vi "Tree_navigation.vi"(8 "error in (no error)":errorcluster, 9 "Tag":string, 10 "Operation":T1(ring), 11 "Script_Tree":refnum<vi>) -> (0 "error out":errorcluster, 2 "Data":string, 3 "Script_Tree 2":refnum<vi>)   [LabVIEW 2024, in "Setting_Screen.lvlib"]
uses:
  Setting_Screen.lvlib
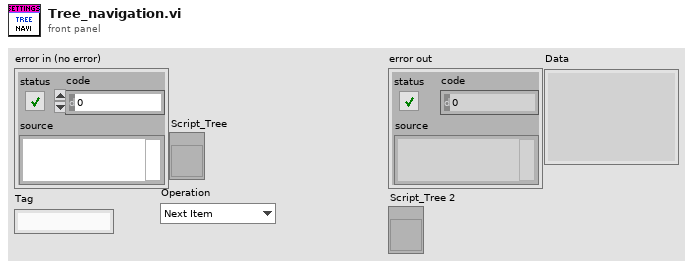
[diagram p1: front panel]
types:
  T1 = enum16{"Next Item", "Previous Item", "Get Child", "Get Parent", "Get Path"}
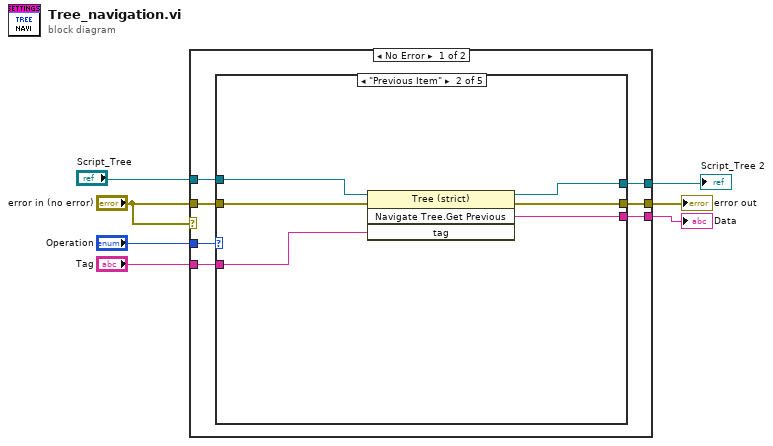
[diagram p0: block diagram]
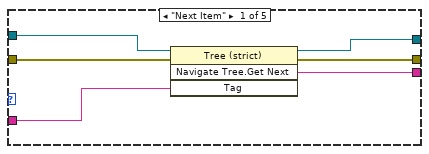
[diagram p2: hidden frame]
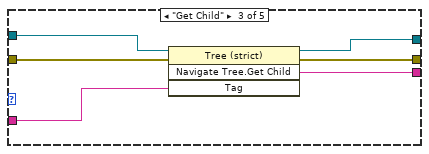
[diagram p3: hidden frame]
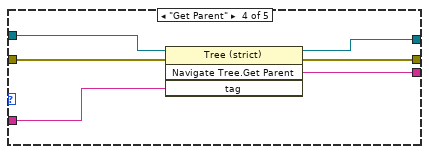
[diagram p4: hidden frame]
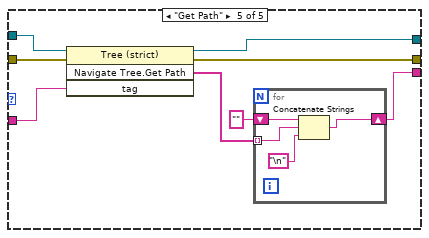
[diagram p5: hidden frame]
diagram:
  n1 = case shown="No Error" "error in (no error)" {
    tunnel: "Operation" -> [w14 _]
    tunnel: "error in (no error)" -> [w13 w51]
    tunnel: "Script_Tree" -> [w12 w52]
    tunnel: [w11 w51] -> w6
    tunnel: [w10 w52] -> w1
    tunnel: [w9 _] -> w5
    tunnel: "Tag" -> [w8 _]
    frame No Error {
      n2 = case shown="\"Previous Item\"" w14 {
        tunnel: w13 -> [w20 w26 w32 w38 w46]
        tunnel: w12 -> [w19 w25 w31 w37 w45]
        tunnel: [w18 w24 w30 w36 w44] -> w10
        tunnel: [w17 w23 w29 w35 w43] -> w11
        tunnel: [w16 w22 w28 w34 w39] -> w9
        tunnel: w8 -> [w15 w21 w27 w33 w42]
        frame "Next Item" {
          n3 = invoke class="Tree (strict)" method="Navigate Tree.Get Next"(reference=w19, error in=w20, "Tag"=w15) -> (reference out=w18:refnum<vi>, error out=w17:errorcluster, "Navigate Tree:Get Next Item"=w16:string)  [unwired: 1 in, 1 out]
        }
        frame "Previous Item" {
          n4 = invoke class="Tree (strict)" method="Navigate Tree.Get Previous"(reference=w25, error in=w26, "tag"=w21) -> (reference out=w24:refnum<vi>, error out=w23:errorcluster, "Navigate Tree:Get Previous"=w22:string)  [unwired: 1 in, 1 out]
        }
        frame "Get Child" {
          n5 = invoke class="Tree (strict)" method="Navigate Tree.Get Child"(reference=w31, error in=w32, "Tag"=w27) -> (reference out=w30:refnum<vi>, error out=w29:errorcluster, "Navigate Tree:Get Child"=w28:string)  [unwired: 1 in, 1 out]
        }
        frame "Get Parent" {
          n6 = invoke class="Tree (strict)" method="Navigate Tree.Get Parent"(reference=w37, error in=w38, "tag"=w33) -> (reference out=w36:refnum<vi>, error out=w35:errorcluster, "Navigate Tree:Get Parent"=w34:string)  [unwired: 1 in, 1 out]
        }
        frame "Get Path" {
          n7 = invoke class="Tree (strict)" method="Navigate Tree.Get Path"(reference=w45, error in=w46, "tag"=w42) -> (reference out=w44:refnum<vi>, error out=w43:errorcluster, "Navigate Tree:Get Path"=w41:string[])  [unwired: 1 in, 1 out]
          n8 = for {
            tunnel: w41 -> [w49] mode=indexing
            shift-right: [w47] -> w39
            shift-left: "" -> [w50]
            n9 = Concatenate Strings(w50, w49, "\n") -> (w47:string)
          }
        }
      }
    }
    frame Error {
    }
  }
  "error out" <- w6
  "Data" <- w5
  "Script_Tree 2" <- w1
